vi "Finalize.vi"(8 "error in":errorcluster, 11 "Shared Resources in":refnum<class "Shared Resources.lvclass">) -> (0 "error out":errorcluster, 3 "Shared Resources out":refnum<class "Shared Resources.lvclass">)   [LabVIEW 2020, in "AIM ARINC 664 Engine.lvlib" / "Implementation.lvlib" / "Shared Resources.lvclass"]
uses:
  Shared Resources.lvclass
  Program Files/National Instruments/LabVIEW 2024/instr.lib/AIM GmbH/_AIM 664/AIM664LV.lvlib
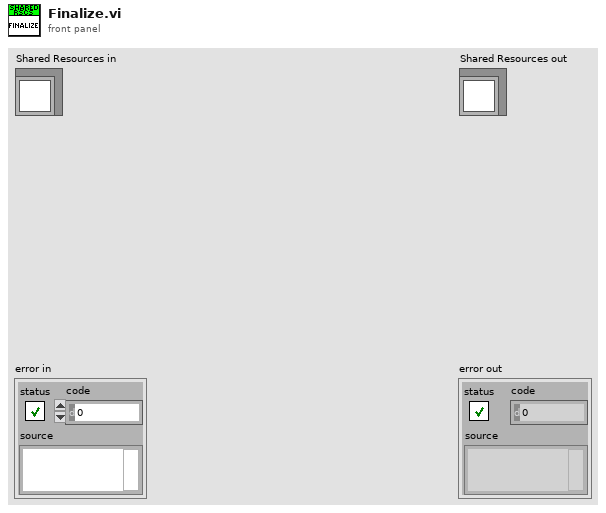
[diagram p1: front panel]
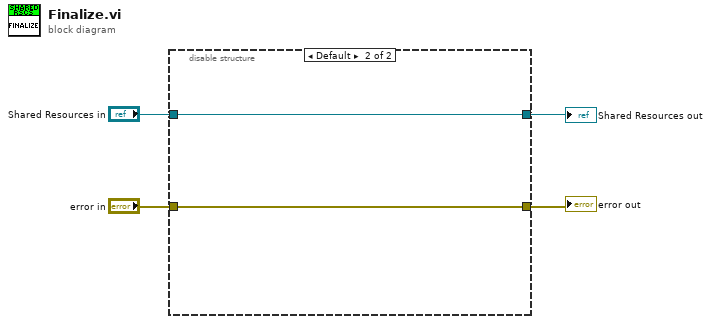
[diagram p0: block diagram]
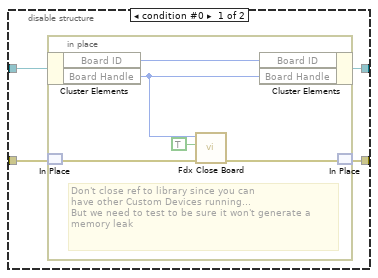
[diagram p2: hidden frame]
diagram:
  n1 = disable-structure shown="Default" {
    disable-tunnel: "error in" -> [w8 w14]
    disable-tunnel: [w7 w14] -> w3
    disable-tunnel: [w6 w15] -> w2
    disable-tunnel: "Shared Resources in" -> [w5 w15]
    frame condition #0 {
      n2 = in-place {
        # "Don't close ref to library since you can\nhave other Custom Devices running...\nBut we need to test to be sure it won't generate a memory leak"
        n3 = in-place-cluster #1(w5) -> ("Board ID"=w13:i32, "Board Handle"=w10:i32)
        n4 = in-place-match #2(w8) -> (w12:errorcluster)
        n5 = call "Fdx Close Board.vi"("error in"=w12, "Force Board Release (F)"=TRUE ("Close reference to library?"), "InstrumentHandle_board in"=w10) -> ("error out"=w11:errorcluster)  [unwired: 8 in]
        n6 = in-place-cluster #1("Board ID"=w13, "Board Handle"=w10) -> (w6:refnum<class "Shared Resources.lvclass">)
        n7 = in-place-match #2(w11) -> (w7:errorcluster)
      }
    }
    frame condition #1 (active) {
    }
  }
  "error out" <- w3
  "Shared Resources out" <- w2
